vi "VariantToProperties.vi"(8 "error in (no error)":errorcluster, 11 "Variant":variant) -> (0 "error out":errorcluster, 3 "Properties":T1[](array[typedef]))   [LabVIEW 2020]
doc: "Converts an array of SLSC properties stored in the SysDef tree into the visual representation for the page."
uses:
  SLSC EDS API/JSON parsing/propertySysDefPage.ctl
  SLSC EDS API/JSON parsing/property.ctl
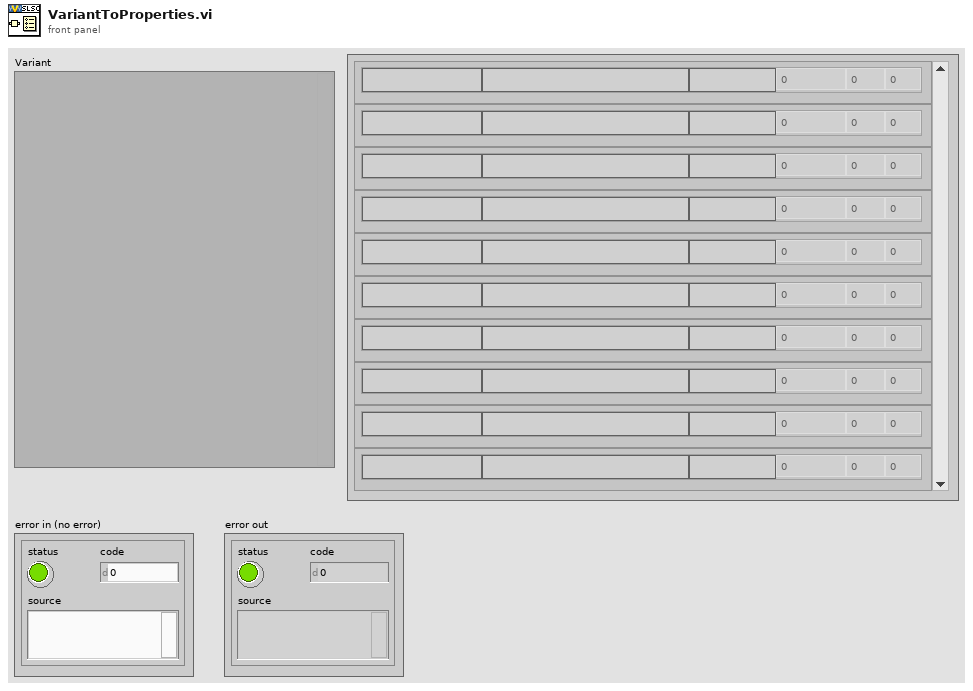
[diagram p1: front panel]
types:
  T1 = typedef "propertySysDefPage.ctl" = cluster{"name":string, "description-en":string, "dataType":string, "value":dbl, "min":dbl, "max":dbl}
  T2 = typedef "property.ctl" = cluster{"name":string, "description-en":string, "documentation-en":string, "dataType":string, "bitfield":string, "access":string, "scale":string, "value":variant, "min":variant, "max":variant, "default value":variant}
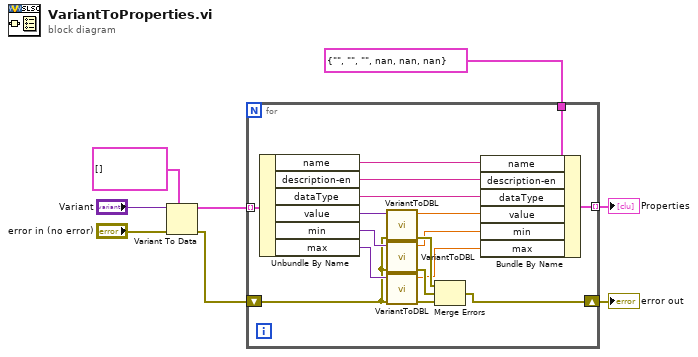
[diagram p0: block diagram]
diagram:
  n1 = Variant To Data(error in="error in (no error)", type=T2[] [] ("properties"), Variant="Variant") -> (data=w2:T2[], error out=w6:errorcluster)
  n2 = for {
    tunnel: w2 -> [w25] mode=indexing
    tunnel: T1 {"name"="", "description-en"="", "dataType"="", "value"=nan, "min"=nan, "max"=nan} ("property") -> [w24]
    tunnel: [w20] -> w3 mode=indexing
    shift-right: [w9] -> w8
    shift-left: w6 -> [w15]
    n3 = Unbundle By Name(w25) -> ("name"=w23:string, "description-en"=w22:string, "dataType"=w21:string, "value"=w19:variant, "min"=w17:variant, "max"=w16:variant)
    n4 = call "VariantToDBL.vi"("error in"=w15, "variant"=w19) -> ("error out"=w13:errorcluster, "data"=w18:dbl)  [unwired: 8 in]
    n5 = call "VariantToDBL.vi"("error in"=w15, "variant"=w17) -> ("error out"=w12:errorcluster, "data"=w11:dbl)  [unwired: 8 in]
    n6 = call "VariantToDBL.vi"("error in"=w15, "variant"=w16) -> ("error out"=w14:errorcluster, "data"=w10:dbl)  [unwired: 8 in]
    n7 = Merge Errors(w13, w12, w14) -> (w9:errorcluster)
    n8 = Bundle By Name(cluster=w24, "name"=w23, "description-en"=w22, "dataType"=w21, "value"=w18, "min"=w11, "max"=w10) -> (w20:T1)
  }
  "Properties" <- w3
  "error out" <- w8
